vi "create_LS372_Data_header_units.vi"() -> (3 "String":string)   [LabVIEW 2018]
uses:
  Instrument_Setup.vi
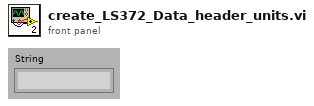
[diagram p1: front panel]
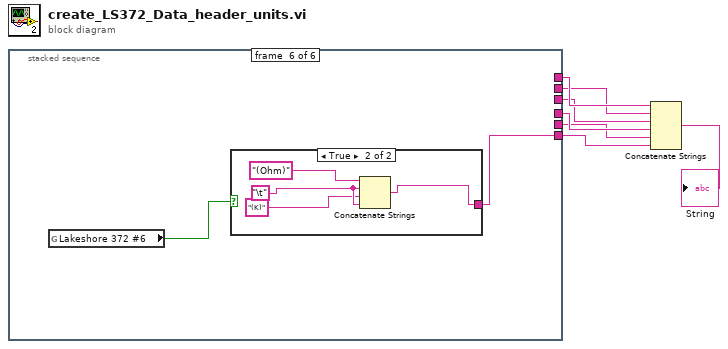
[diagram p0: block diagram]
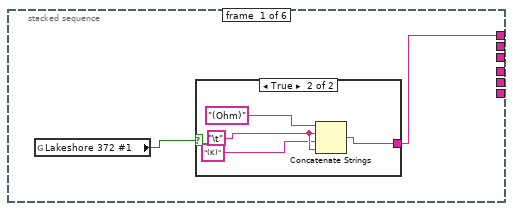
[diagram p2: hidden frame]
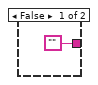
[diagram p3: hidden frame]
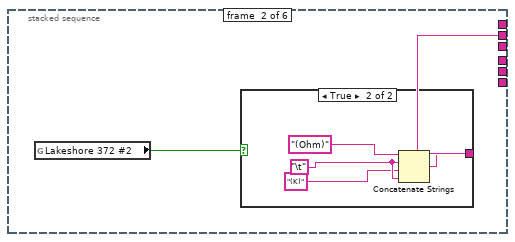
[diagram p4: hidden frame]
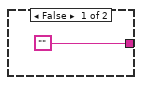
[diagram p5: hidden frame]
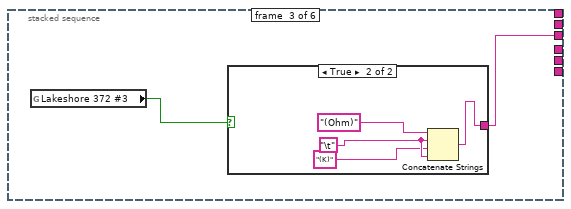
[diagram p6: hidden frame]
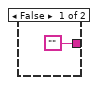
[diagram p7: hidden frame]
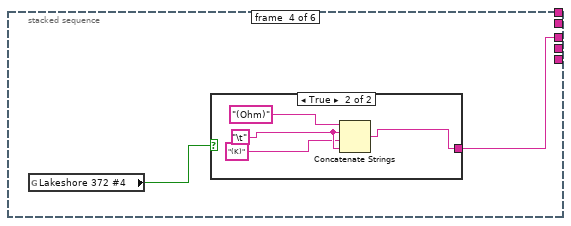
[diagram p8: hidden frame]
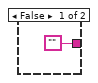
[diagram p9: hidden frame]
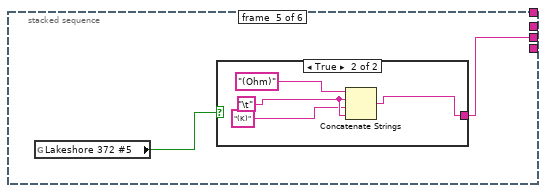
[diagram p10: hidden frame]
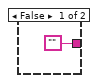
[diagram p11: hidden frame]
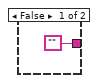
[diagram p12: hidden frame]
diagram:
  n1 = stacked-sequence {
    tunnel: [w8 _ _ _ _ _] -> w7
    tunnel: [_ w15 _ _ _ _] -> w6
    tunnel: [_ _ w22 _ _ _] -> w5
    tunnel: [_ _ _ w29 _ _] -> w4
    tunnel: [_ _ _ _ w36 _] -> w2
    tunnel: [_ _ _ _ _ w43] -> w1
    frame #0 {
      n2 = global read "Instrument_Setup.vi" "Lakeshore 372 #1"() -> (w9:bool)
      n3 = case shown="True" w9 {
        tunnel: ["" w11] -> w8
        frame False {
        }
        frame True {
          w13 = "\t"
          n4 = Concatenate Strings("(Ohm)", w13, "(K)", w13) -> (w11:string)
        }
      }
    }
    frame #1 {
      n5 = global read "Instrument_Setup.vi" "Lakeshore 372 #2"() -> (w16:bool)
      n6 = case shown="True" w16 {
        tunnel: ["" w18] -> w15
        frame False {
        }
        frame True {
          w20 = "\t"
          n7 = Concatenate Strings("(Ohm)", w20, "(K)", w20) -> (w18:string)
        }
      }
    }
    frame #2 {
      n8 = global read "Instrument_Setup.vi" "Lakeshore 372 #3"() -> (w23:bool)
      n9 = case shown="True" w23 {
        tunnel: ["" w25] -> w22
        frame False {
        }
        frame True {
          w27 = "\t"
          n10 = Concatenate Strings("(Ohm)", w27, "(K)", w27) -> (w25:string)
        }
      }
    }
    frame #3 {
      n11 = global read "Instrument_Setup.vi" "Lakeshore 372 #4"() -> (w30:bool)
      n12 = case shown="True" w30 {
        tunnel: ["" w32] -> w29
        frame False {
        }
        frame True {
          w34 = "\t"
          n13 = Concatenate Strings("(Ohm)", w34, "(K)", w34) -> (w32:string)
        }
      }
    }
    frame #4 {
      n14 = global read "Instrument_Setup.vi" "Lakeshore 372 #5"() -> (w37:bool)
      n15 = case shown="True" w37 {
        tunnel: ["" w39] -> w36
        frame False {
        }
        frame True {
          w41 = "\t"
          n16 = Concatenate Strings("(Ohm)", w41, "(K)", w41) -> (w39:string)
        }
      }
    }
    frame #5 {
      n17 = global read "Instrument_Setup.vi" "Lakeshore 372 #6"() -> (w44:bool)
      n18 = case shown="True" w44 {
        tunnel: ["" w46] -> w43
        frame False {
        }
        frame True {
          w48 = "\t"
          n19 = Concatenate Strings("(Ohm)", w48, "(K)", w48) -> (w46:string)
        }
      }
    }
  }
  n20 = Concatenate Strings(w7, w6, w5, w4, w2, w1) -> (→"String":string)
